vi "图片自适应居中.vi"(8 "图片框引用":refnum<vi>, 11 "图片路径":path=path "E:/Program Files (x86)/National Instruments/LabVIEW 2013/data/历史照片/迷你面板.png") -> (0 "错误输出":errorcluster)   [LabVIEW 2017]
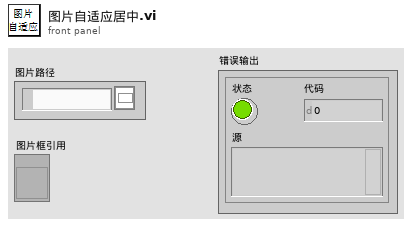
[diagram p1: front panel]
types:
  T1 = typedef "imagedata.ctl" = cluster{"image type":i32, "image depth":i32, "image":u8[], "mask":u8[], "colors":u32[], "Rectangle":cluster{"left":i16, "top":i16, "right":i16, "bottom":i16}}
  T2 = typedef "LVBoundsTypeDef.ctl" = cluster{"Width":u32, "Height":u32}
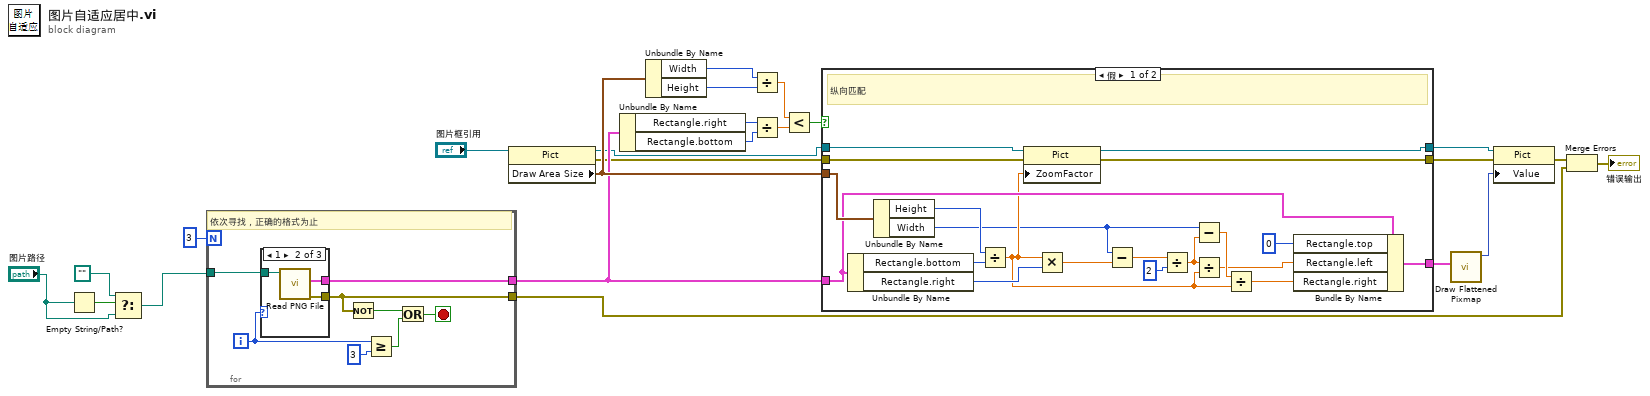
[diagram p0: block diagram]
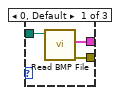
[diagram p2: hidden frame]
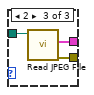
[diagram p3: hidden frame]
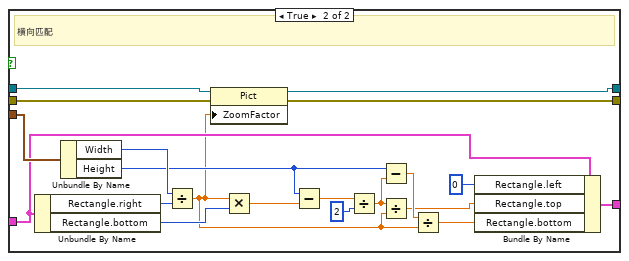
[diagram p4: hidden frame]
diagram:
  n1 = Empty String/Path?(string/path="图片路径") -> (empty?=w4:bool)
  n2 = Select(t=path "", s=w4, f="图片路径") -> (s? t:f=w1:path)
  n3 = for {
    N: 3 -> [_]
    tunnel: w1 -> [w32]
    tunnel: [w26] -> w14
    tunnel: [w25] -> w5
    i -> [w28]
    stop <- w30 stop-if-true
    # "依次寻找，正确的格式为止"
    n4 = case shown="1" w28 {
      tunnel: w32 -> [w35 w38 w41]
      tunnel: [w34 w37 w40] -> w25
      tunnel: [w33 w36 w39] -> w26
      frame 0, Default {
        n5 = call <vilib>:"Read BMP File.vi"("path to BMP file"=w35) -> ("error out"=w34:errorcluster, "image data"=w33:T1)  [unwired: 8 in, 1 out]
      }
      frame 1 {
        n6 = call <vilib>:"Read PNG File.vi"("path to PNG file"=w38) -> ("error out"=w37:errorcluster, "image data"=w36:T1)  [unwired: 8 in, 1 out]
      }
      frame 2 {
        n7 = call <vilib>:"Read JPEG File.vi"("path to JPEG file"=w41) -> ("error out"=w40:errorcluster, "image data"=w39:T1)  [unwired: 8 in, 1 out]
      }
    }
    n8 = Not(x=w25) -> (.not. x?=w31:bool)
    n9 = Greater Or Equal?(x=w28, y=3 ("x")) -> (x >= y?=w27:bool)
    n10 = Or(x=w31, y=w27) -> (x .or. y?=w30:bool)
  }
  n11 = property on="属性节点" class="Pict"(reference="图片框引用") -> (reference out=w12:refnum<vi>, error out=w11:errorcluster, "Draw Area Size"=w17:T2)  [unwired: 1 in]
  n12 = Unbundle By Name(w14) -> ("Rectangle.right"=w19:i16, "Rectangle.bottom"=w18:i16)
  n13 = Unbundle By Name(w17) -> ("Width"=w21:u32, "Height"=w20:u32)
  n14 = Divide(x=w21, y=w20) -> (x/y=w24:dbl)
  n15 = Divide(x=w19, y=w18) -> (x/y=w23:dbl)
  n16 = Less?(x=w24, y=w23) -> (x < y?=w22:bool)
  n17 = case shown="假" w22 {
    tunnel: w17 -> [w61 w81]
    tunnel: w14 -> [w52 w72]
    tunnel: [w56 w76] -> w16
    tunnel: w12 -> [w45 w65]
    tunnel: w11 -> [w44 w64]
    tunnel: [w43 w63] -> w8
    tunnel: [w42 w62] -> w9
    frame False {
      # "纵向匹配"
      n18 = Unbundle By Name(w52) -> ("Rectangle.bottom"=w55:i16, "Rectangle.right"=w54:i16)
      n19 = Unbundle By Name(w61) -> ("Height"=w60:u32, "Width"=w46:u32)
      n20 = Divide(x=w60, y=w55) -> (x/y=w48:dbl)
      n21 = property on="属性节点" class="Pict"(reference=w45, error in=w44, "ZoomFactor"=w48) -> (reference out=w42:refnum<vi>, error out=w43:errorcluster)
      n22 = Multiply(x=w48, y=w54) -> (x*y=w53:dbl)
      n23 = Subtract(x=w46, y=w53) -> (x-y=w58:dbl)
      n24 = Divide(x=w58, y=u32 2) -> (x/y=w47:dbl)
      n25 = Subtract(x=w46, y=w47) -> (x-y=w51:dbl)
      n26 = Divide(x=w47, y=w48) -> (x/y=w50:dbl)
      n27 = Divide(x=w51, y=w48) -> (x/y=w49:dbl)
      n28 = Bundle By Name(cluster=w52, "Rectangle.top"=i16 0 ("Rectangle.left"), "Rectangle.left"=w50, "Rectangle.right"=w49) -> (w56:T1)
    }
    frame True {
      # "横向匹配"
      n29 = Unbundle By Name(w72) -> ("Rectangle.right"=w75:i16, "Rectangle.bottom"=w74:i16)
      n30 = Unbundle By Name(w81) -> ("Width"=w80:u32, "Height"=w71:u32)
      n31 = Divide(x=w80, y=w75) -> (x/y=w66:dbl)
      n32 = property on="属性节点" class="Pict"(reference=w65, error in=w64, "ZoomFactor"=w66) -> (reference out=w62:refnum<vi>, error out=w63:errorcluster)
      n33 = Multiply(x=w66, y=w74) -> (x*y=w73:dbl)
      n34 = Subtract(x=w71, y=w73) -> (x-y=w78:dbl)
      n35 = Divide(x=w78, y=u32 2) -> (x/y=w69:dbl)
      n36 = Subtract(x=w71, y=w69) -> (x-y=w70:dbl)
      n37 = Divide(x=w69, y=w66) -> (x/y=w68:dbl)
      n38 = Divide(x=w70, y=w66) -> (x/y=w67:dbl)
      n39 = Bundle By Name(cluster=w72, "Rectangle.left"=i16 0, "Rectangle.top"=w68, "Rectangle.bottom"=w67) -> (w76:T1)
    }
  }
  n40 = call <vilib>:"Draw Flattened Pixmap.vi"("image data"=w16) -> ("new picture"=w10:picture)  [unwired: 8 in]
  n41 = property on="属性节点" class="Pict"(reference=w9, error in=w8, "Value"=w10) -> (error out=w7:errorcluster)  [unwired: 1 out]
  n42 = Merge Errors(w7, w5) -> (→"错误输出":errorcluster)
